vi "VI Linearisierung v2.vi"() -> ()   [LabVIEW 2020, in "Linearisierung v2.lvlib"] (continued)
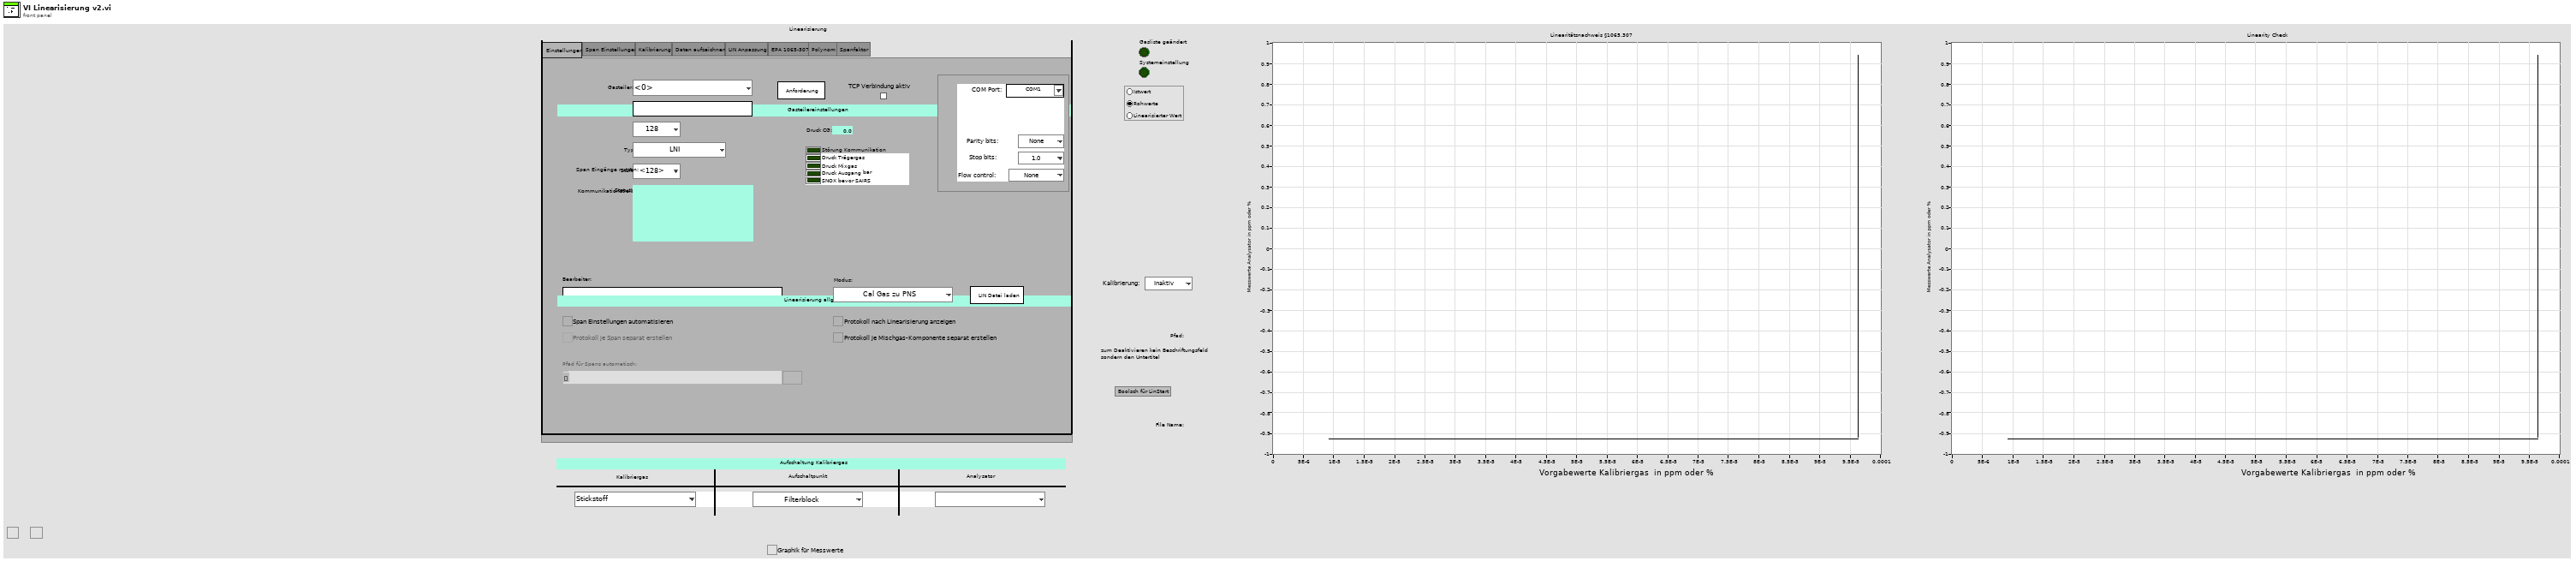
[diagram p1: front panel]
types:
  T1 = typedef "Checkbox(boolsch).ctl" = bool
  T2 = typedef "Linearisierung v2.lvlib/EPA Optionsfeld.ctl" = enum32{"Istwert", "Rohwert", "Linearisierter Wert"}
  T3 = typedef "EPA 1065.lvlib/T90 Test 1065-308.lvlib/Auswahl.ctl" = bool
  T4 = typedef "Button.ctl" = bool
  T5 = typedef "Linearisierung v2.lvlib/Kalibrieroption.ctl" = u16
  T6 = typedef "CalGas Aufschaltung.lvlib/Aufschaltung CalGas_ANZEIGE.ctl" = cluster{"Kalibriergas":T7, "Aufschaltpunkt":T7, "Analysator":T7}
  T7 = typedef "Auswahlfeld.ctl" = u16
  T8 = enum32{"Einstellungen", "Span Einstellungen", "HovaCAL Interface", "Kalibrierung", "Daten aufzeichnen", "LIN Anpassung", "EPA 1065-307", "Polynomkoeffizienten", "HovaCal Einstellungen", "Spanfaktor"}
  T9 = typedef "Pfad-Eingabefeld.ctl" = path
  T10 = typedef "CalGas Aufschaltung.lvlib/Lin Modus.ctl" = u16
  T11 = typedef "System Einstellungen V2.lvlib/Gasteiler Auswahl.ctl" = u16
  T12 = typedef "String - Eingabefeld.ctl" = string
  T13 = typedef "Linearisierung v2.lvlib/Gasteiler.lvlib/RS232.ctl" = cluster{"VISA Resource Name":refnum<visa-resource-name>, "Baud Rate":u32, "data bits":u16, "parity":u16, "stop bits":u16, "flow control":u16}
  T14 = typedef "Zahlen-Ausgabefeld.ctl" = sgl
  T15 = typedef "Linearisierung v2.lvlib/GasteilerType.ctl" = u16
  T16 = typedef "Linearisierung v2.lvlib/Gasteiler.lvlib/Gasteiler Stufen.ctl" = u16
  T17 = typedef "Linearisierung v2.lvlib/Gasteiler.lvlib/Gasteiler Fehler.ctl" = cluster{"Pressure carrier gas":bool, "Pressure diluted gas":bool, "Outlet Pressure":bool, "SNOX before SAIR":bool}
  T18 = enum32{"SPAN  1", "SPAN  2", "SPAN  3", "SPAN  4", "SPAN  5", "SPAN  6", "SPAN  7", "SPAN  8", "SPAN  9", "SPAN  10"}
  T19 = typedef "Linearisierung v2.lvlib/SpanEinstellungen.lvlib/SpanInletCluster.ctl" = cluster{"Span Inlet Active":T20, "Analysator":T21, "Konfig Gasflasche":T20, "Gasflasche":T22, "Gasflaschen Nr.:":string, "Ablaufdatum":timestamp, "Komponenten":T23, "Zeitdauer Stufen":sgl, "Max Fehler":sgl, "Anzahl Stufen":sgl, "Trägergas":T26, "zusätzliche Zeitdauer Erster Punkt":sgl}
  T20 = typedef "System Einstellungen V2.lvlib/Konfig Gasflasche.ctl" = bool
  T21 = typedef "System Einstellungen V2.lvlib/Analysatoren.ctl" = string
  T22 = typedef "System Einstellungen V2.lvlib/Gasflasche Auswahl.ctl" = u16
  T23 = typedef "Linearisierung v2.lvlib/SpanEinstellungen.lvlib/Komponentencluster mit Formel.ctl" = cluster{"Komponente 1":T24, "Komponente 2":T24, "Komponente 3":T24, "Komponente 4":T24, "Komponente 5":T24}
  T24 = typedef "Linearisierung v2.lvlib/SpanEinstellungen.lvlib/Komponentenauswahl mit Formel.ctl" = cluster{"Komponente:":u16, "Summenformel":T12, "Konzentration IST":dbl, "Einheit":T25, "Genauigkeit":dbl}
  T25 = typedef "Linearisierung v2.lvlib/SpanEinstellungen.lvlib/Einheit.ctl" = enum16{"ppm", "%"}
  T26 = typedef "System Einstellungen V2.lvlib/Traegergas.ctl" = string
  T27 = typedef "Linearisierung v2.lvlib/Gasteiler.lvlib/Stufen Tabelle.ctl" = string[][]
  T28 = typedef "Linearisierung v2.lvlib/Parameterkontrolle.ctl" = string[]
  T29 = typedef "Linearisierung v2.lvlib/Gasteiler.lvlib/HovaCAL_Interface.lvlib/Controls.lvlib/Pumpen Parameter Anzeige Eingabe.ctl" = cluster{"Reagent":T30, "concentratio mode":T31, "Molarity":dbl, "density":dbl, "syringe":dbl, "pumpe_a":dbl}[]
  T30 = typedef "Linearisierung v2.lvlib/Gasteiler.lvlib/HovaCAL_Interface.lvlib/Controls.lvlib/Reagent Anzeige.ctl" = i32
  T31 = typedef "Linearisierung v2.lvlib/Gasteiler.lvlib/HovaCAL_Interface.lvlib/Controls.lvlib/Pump Concentration Mode Anzeige.ctl" = i32
  T32 = typedef "Linearisierung v2.lvlib/Gasteiler.lvlib/HovaCAL_Interface.lvlib/Controls.lvlib/Pump state.ctl" = cluster{"Run":bool}
  T33 = typedef "Linearisierung v2.lvlib/Gasteiler.lvlib/HovaCAL_Interface.lvlib/Controls.lvlib/Flow Einstellung.ctl" = cluster{"HovaCAL Flow Input Cluster":dbl}
  T34 = typedef "Linearisierung v2.lvlib/Gasteiler.lvlib/HovaCAL_Interface.lvlib/Controls.lvlib/Flow Anzeige.ctl" = cluster{"Actual Flow":dbl}
  T35 = typedef "Linearisierung v2.lvlib/Gasteiler.lvlib/HovaCAL_Interface.lvlib/Controls.lvlib/Pumpen Parameter Anzeige.ctl" = cluster{"Reagent":T30, "concentratio mode":T31, "Molarity":dbl, "density":dbl, "syringe":dbl, "pumpe_a":dbl}[]
  T36 = typedef "Linearisierung v2.lvlib/Gasteiler.lvlib/HovaCAL_Interface.lvlib/Controls.lvlib/Pumpe Modus Anzeige.ctl" = cluster{"running?":bool, "dry mode":T37, "control mode":T38}
  T37 = typedef "Linearisierung v2.lvlib/Gasteiler.lvlib/HovaCAL_Interface.lvlib/Controls.lvlib/Pump Dry Mode Anzeige.ctl" = i32
  T38 = typedef "Linearisierung v2.lvlib/Gasteiler.lvlib/HovaCAL_Interface.lvlib/Controls.lvlib/Pump Control Mode Anzeige.ctl" = u32
  T39 = typedef "Linearisierung v2.lvlib/Gasteiler.lvlib/HovaCAL_Interface.lvlib/Controls.lvlib/Pumpe Status Anzeige.ctl" = cluster{"running?":bool, "Speed":dbl[]}
  T40 = typedef "Linearisierung v2.lvlib/Gasteiler.lvlib/HovaCAL_Interface.lvlib/Controls.lvlib/Pumpe MassenFluss Anzeige.ctl" = cluster{"reagent mf SP":dbl, "reagent mf":dbl, "water mf SP":dbl, "water mf":dbl, "water/reagent mf SP":dbl, "water/reagent mf":dbl}[]
  T41 = typedef "Linearisierung v2.lvlib/Gasteiler.lvlib/HovaCAL_Interface.lvlib/Controls.lvlib/Grenzen Anzeige.ctl" = cluster{"flow":dbl[], "temp":dbl[]}
  T42 = typedef "Linearisierung v2.lvlib/Gasteiler.lvlib/HovaCAL_Interface.lvlib/Controls.lvlib/Temp Sollwerte Anzeige.ctl" = dbl[]
  T43 = typedef "Linearisierung v2.lvlib/Gasteiler.lvlib/HovaCAL_Interface.lvlib/Controls.lvlib/Temp Ausgang Anzeige.ctl" = cluster{"temp 2":dbl, "temp":dbl, "humidity":dbl}[]
  T44 = typedef "Linearisierung v2.lvlib/Gasteiler.lvlib/HovaCAL_Interface.lvlib/Controls.lvlib/MFC Einstellungen.ctl" = cluster{"Input Concentration":dbl, "Output Setpoint":dbl}
  T45 = typedef "Linearisierung v2.lvlib/Gasteiler.lvlib/HovaCAL_Interface.lvlib/Controls.lvlib/MFC Output.ctl" = cluster{"output concentration":dbl, "output concentration dry":dbl, "flow actual":dbl, "flow expected":dbl}
  T46 = typedef "Linearisierung v2.lvlib/Gasteiler.lvlib/HovaCAL_Interface.lvlib/Controls.lvlib/MFC Konfiguration.ctl" = cluster{"MFC Gasauswahl":u16}
  T47 = typedef "Linearisierung v2.lvlib/Gasteiler.lvlib/HovaCAL_Interface.lvlib/Controls.lvlib/Pumpen Output.ctl" = cluster{"reagent conc":dbl, "reagent conc dry":dbl, "water conc":dbl, "water conc dry":dbl, "speed":dbl}
  T48 = typedef "String - Ausgabefeld.ctl" = string
  T49 = typedef "Linearisierung v2.lvlib/Gasnumber.ctl" = u8
  T50 = typedef "Linearisierung v2.lvlib/Gasteiler.lvlib/HovaCAL_Interface.lvlib/Controls.lvlib/Info Cluster Anzeige.ctl" = cluster{"device":string, "version":string, "number of mfc":i32, "number of pumps":i32, "number of temp controllers":i32, "number of mfs":i32, "number of balances":i32}
  T51 = typedef "Linearisierung v2.lvlib/Gasteiler.lvlib/HovaCAL_Interface.lvlib/Controls.lvlib/MFC Flow Anzeige.ctl" = cluster{"min flow":dbl, "max flow":dbl}[]
  T52 = typedef "Linearisierung v2.lvlib/Polynomkoeffizientenanzeige.ctl" = cluster{"Offset":dbl, "O.1":dbl, "O. 2":dbl, "O. 3":dbl, "O. 4":dbl}
  T53 = typedef "Linearisierung v2.lvlib/Ausgabetabelle.ctl" = string[][]
  T54 = typedef "Linearisierung v2.lvlib/Eingabetabelle.ctl" = string[][]
  T55 = typedef "Linearisierung v2.lvlib/Auswahl Polynom Ordnung.ctl" = enum16{"autom.", "raw", "actual", "1", "2", "3", "4"}
  T56 = typedef "Linearisierung v2.lvlib/LIN Ausgabetabelle.ctl" = string[][]
  T57 = typedef "Linearisierung v2.lvlib/AktivArray.ctl" = T58[]
  T58 = typedef "Linearisierung v2.lvlib/AktivButton.ctl" = bool
  T59 = typedef "Linearisierung v2.lvlib/Linearity verification 1065-307.lvlib/Condition.ctl" = u16
  T60 = typedef "Linearisierung v2.lvlib/EPA Ausgabetabelle.ctl" = string[][]
  T61 = typedef "Linearisierung v2.lvlib/Gasteiler.lvlib/HovaCal.lvlib/AutoLin Hovacal.ctl" = enum32{"Keine Auswahl", "Optionsauswahl 1", "Optionsauswahl 2"}
  T62 = typedef "Linearisierung v2.lvlib/Gasteiler.lvlib/HovaCal.lvlib/Dynamsiche_Werte.ctl" = cluster{"Durchfluss":dbl, "Drehzahl":dbl, "Wasserkonz.":dbl, "Ist - Temp":dbl, "Ist Konz 1":dbl, "Ist Konz 2":dbl}
  T63 = typedef "Linearisierung v2.lvlib/Gasteiler.lvlib/HovaCal.lvlib/Gase.ctl" = cluster{"Trägergas":u16, "Komponente 1":u16, "Komponente 2":u16}
  T64 = typedef "Linearisierung v2.lvlib/Gasteiler.lvlib/HovaCal.lvlib/Betriebsdaten.ctl" = cluster{"Gesamtdurchfluss":dbl, "Eingangskonzentration \nTrägergas":dbl, "Eingangskonzentration\nKomponente 1":dbl, "Eingangskonzentration \nKomponente 2":dbl, "Ausgangskonzentration \nKomponente 1 ":dbl, "Ausgangskonzentration\nKomponente 2":dbl, "l/min -> ml/min":bool, "N2 %->ppm":bool, "Komp1 ppm->%":bool, "Komp2ppm->%":bool, "Sollkomp1ppm->%":bool, "Sollkomp2ppm->%":bool}
  T65 = typedef "Linearisierung v2.lvlib/Gasteiler.lvlib/HovaCal.lvlib/Vaporizer.ctl" = cluster{"Pumpe Ein/Aus":dbl, "Wasser / Reagent":dbl, "Reagent dry / wet":dbl, "Reagent":dbl, "min. Temperatur\n160 °C":dbl, "Solltemperatur":dbl, "Wasserkonzentration\nSoll":dbl}
  T66 = enum8{"Enabled", "Disabled", "Disabled and Grayed Out"}
  T67 = typedef "Linearisierung v2.lvlib/SpanEinstellungen.lvlib/Aktion FGV SPAN Stufentabellen.ctl" = enum16{"lesen", "schreiben", "init"}
  T68 = typedef "Linearisierung v2.lvlib/Protokoll.lvlib/Aktion LIN Polynom Ordnung ode Aktiv Changes für Postprocessing.ctl" = enum16{"lesen", "schreiben", "init", "init initial"}
  T69 = cluster{"active SPAN Idx":i32, "active Component Index":i32}
  T70 = typedef "Linearisierung v2.lvlib/Protokoll.lvlib/Aktion LIN Polynom Ordnung je Komponente für Protokoll.ctl" = enum16{"lesen", "schreiben", "init", "schreiben viewonly", "init initial"}
  T71 = typedef "Linearisierung v2.lvlib/SpanEinstellungen.lvlib/Aktion FGV Post Processing.ctl" = enum16{"lesen", "set ref", "init", "reset", "enable", "disable", "filenames", "active", "comp", "filename index", "next", "first", "abort", "show", "same"}
  T72 = typedef "Linearisierung v2.lvlib/Gasteiler.lvlib/Aktion FGV Gasteilerliste laden.ctl" = enum16{"lesen", "laden", "speichern", "Liste erstellen", "Formel ändern", "Gas vereinzeln"}
  T73 = typedef "Linearisierung v2.lvlib/SpanEinstellungen.lvlib/Aktion FGV SPAN Verriegelung.ctl" = enum16{"lesen", "setrefs", "setcomp", "lock", "unlock", "Set Save EPA redirect", "Reset Save EPA redirect", "Set Postprocessing PDF", "Reset Postprocessing PDF", "Set Start Postprocessing PDF", "Reset Start Postprocessing PDF"}
  T74 = typedef "Linearisierung v2.lvlib/SpanEinstellungen.lvlib/Aktion FGV Spans abarbeiten.ctl" = enum16{"lesen", "idle", "start", "next", "comp", "init", "running", "abort"}
  T75 = typedef "Linearisierung v2.lvlib/SpanEinstellungen.lvlib/Aktion FGV SpanEinstellungen.ctl" = enum16{"lesen", "schreiben", "laden", "speichern", "RegisterRef", "automatisch", "init", "PDF Params", "Punkte umkehren"}
  T76 = typedef "System Einstellungen V2.lvlib/Aktion FGV Gasbottledefinition.ctl" = enum16{"lesen", "schreiben", "löschen", "laden", "speichern", "exportieren", "importieren"}
  T77 = typedef "Linearisierung v2.lvlib/SpanEinstellungen.lvlib/Aktion FGV Komponentenreferenz verwalten.ctl" = enum16{"Referenzen init", "lesen", "Referenzen schließen", "Ring beschreiben", "MFC fix Werte setzen"}
  T78 = typedef "FT-IR.lvlib/FGV FT-IR Gasliste Aktionen.ctl" = enum16{"lesen", "Gasliste FT-IR", "Gasliste ausgelesen", "laden", "speichern", "löschen"}
  T79 = typedef "Linearisierung v2.lvlib/Gasteiler.lvlib/HovaCAL_Interface.lvlib/Kommunikation.lvlib/Aktion_FGV_HovaCAL_Interface_Kommandos.ctl" = enum16{"lesen", "verarbeiten", "hinzufügen", "on top", "init", "sammeln", "freigeben", "connected"}
  T80 = typedef "Linearisierung v2.lvlib/Gasteiler.lvlib/HovaCAL_Interface.lvlib/Kommunikation.lvlib/Aktion_FGV_HovaCAL_Interface_GetData.ctl" = enum16{"lesen", "SystemInfo", "MFC Info", "actual Values", "Limits", "first contact", "reset after read"}
  T81 = typedef "Linearisierung v2.lvlib/Gasteiler.lvlib/HovaCAL_Interface.lvlib/Kommunikation.lvlib/Aktion_FGV_HovaCAL_Interface_SetData.ctl" = enum16{"lesen", "Konzentrationen", "Pumpen Parameter", "Pumpe Konzentration", "Pumpe run", "Temperaturen", "Fluss", "Limits", "init"}
  T82 = typedef "Linearisierung V2.lvlib/Aktion FGV Rohmesswerte sammeln.ctl" = enum16{"lesen", "schreiben", "löschen", "Sollwert HovaCal"}
  T83 = typedef "Linearisierung v2.lvlib/Aktion FGV Stoerungen sammeln und auswerten.ctl" = enum16{"init", "lesen", "error", "prüfen", "reset error", "abbrechen", "fortsetzen", "neustart", "Bedientasten reset"}
  T84 = typedef "Linearisierung v2.lvlib/Gasteiler.lvlib/Aktionen FGV Gasteiler Daten.ctl" = enum16{"lesen", "Gasteiler Daten", "Seriellen Param.", "MB-Endwert", "laden", "speichern", "Anforderung", "TCP", "Aufzeichnung Start"}
  T85 = typedef "FT-IR.lvlib/Spanfaktor.lvlib/Aktion FGV Span.ctl" = enum16{"lesen", "Span", "Seite aktiv", "Offset", "FGV aktualisiert", "Aktualisierung aufheben"}
  T86 = typedef "CalGas Aufschaltung.lvlib/FGV CalGas Aktionen.ctl" = enum16{"lesen", "Analysator Auswahl", "Def.CalGas", "Aufschaltung CalGas", "laden", "speichern", "KAL extrahieren"}
  T87 = typedef "Linearisierung v2.lvlib/LinV2 Registerkarten.ctl" = enum32{"Einstellungen", "HovaCAL Interface", "Kalibrierung", "Daten aufzeichnen", "LIN Anpassung", "EPA 1065-307", "Polynomkoeffizienten", "HovaCal Einstellungen", "Spanfaktor"}
  T88 = typedef "Linearisierung v2.lvlib/Gasteiler.lvlib/HovaCal.lvlib/Aktion_FGV_Betriebsdaten.ctl" = enum16{"Lesen", "Sollwerte schreiben", "Sollwerte lesen", "Gase schreiben", "Gase lesen", "Dynamische Werte", "GaseRef", "Gase aendern"}
  T89 = typedef "Linearisierung v2.lvlib/Gasteiler.lvlib/Gasteiler Type.ctl" = enum16{"LNI Digital", "LNI Analoge", "AVL GDU ", "Horiba GDC", "HovaCal"}
  T90 = typedef "Linearisierung v2.lvlib/Aktion Lin Daten aufarbeiten.ctl" = enum16{"lesen", "Protkolldaten", "speichern", "laden", "EPA auswerten", "Tabelle schreiben", "Lin auswerten", "Tab init", "Stufentabelle", "EPA aktiviert", "Nachbehandlung laden", "Tabelle löschen", "Istwerte löschen", "Zeile löschen", "Zeile einfügen", "LIN aktiviert", "LIN/EPA aktiv laden", "EGAK Tab", "LIN übernehmen", "Tab init ohne Stufen"}
  T91 = typedef "Linearisierung v2.lvlib/Gasteiler.lvlib/HovaCAL_Interface.lvlib/Kommunikation.lvlib/Aktion FGV HovaCAL Interface Autolin.ctl" = enum16{"lesen", "schreiben", "MFC Komponente fix setzen", "init"}
  T92 = typedef "Linearisierung v2.lvlib/Gasteiler.lvlib/Aktion FGV Daten Abholung uebergebenctl.ctl" = enum16{"lesen", "schreiben", "Anzeigebit löschen", "Status hinzufügen"}
  T93 = typedef "Linearisierung v2.lvlib/Gasteiler.lvlib/Aktion FGV Gasteiler Korrektur.ctl" = enum16{"lesen", "schreiben", "laden", "speichern", "B-nr und Gültig", "Gasteilernr.", "Vereinzeln", "aktiv"}
  T94 = typedef "Linearisierung v2.lvlib/Aktionen Polynom Daten speichern.ctl" = enum16{"lesen", "laden", "speichern", "schreiben", "schreiben alle", "Liste erstellen", "aktivieren", "deaktivieren", "aktiv abfragen"}
  T95 = typedef "Linearisierung v2.lvlib/Gasteiler.lvlib/HovaCal.lvlib/Aktion_FGV_Kom.ctl" = enum16{"Initialisieren", "Betriebsparameter", "Gase", "Vaporizer", "Dynamische Werte", "Beenden", "Com ändern", "Gase init"}
  T96 = typedef "Linearisierung v2.lvlib/Gasteiler.lvlib/HovaCAL_Interface.lvlib/Kommunikation.lvlib/Aktion_FGV_HovaCAL_Interface_Kommunikation.ctl" = enum16{"Initialisieren", "Set Konzentrationen", "Set Gase", "Set Limits", "Get Dynamische Werte", "Beenden", "Com ändern", "Get Gase init", "Pause", "Get Gasteiler Infos", "Get MFC Infos", "Set Pumpen Parameter", "Set Pumpe Konzenration", "Set Pumpe run", "Set Temperaturen", "Set Fluss", "Get Gase", "Get Limits", "Get Dynamische Werte 1", "Get Dynamische Werte 2"}
  T97 = typedef "PDF Interface.lvlib/PDF Interface Helper.lvlib/PDFResultPictures.ctl" = cluster{"Yes Ctl Refnum":refnum<vi>, "No Ctl Refnum":refnum<vi>}
  T98 = typedef "Sprachverwaltung.lvlib/FGV Aktion Tabelle zerlegen.ctl" = enum16{"laden", "vereinzeln", "speichern"}
  T99 = typedef "FT-IR.lvlib/Aktionen EVID-Codes.ctl" = enum16{"lesen", "setzen", "laden", "speichern", "1Hz/5Hz", "Smoothing", "Rolling Average"}
  T100 = typedef "LVRowAndColumnTypeDef.ctl" = cluster{"Row":i32, "Column":i32}
  T101 = cluster{"File Name LIN":refnum<vi>, "EPA Filename":refnum<vi>}
  T102 = cluster{"LIN Filename override":refnum<vi>, "EPA Filename override":refnum<vi>}
  T103 = cluster{"Spanfactor":refnum<vi>, "Offset":refnum<vi>, "Polynom":refnum<vi>}
  T104 = cluster{"Hauptregisterkarte":refnum<vi>, "SpanRegister":refnum<vi>}
  T105 = typedef "System Einstellungen V2.lvlib/Gasflasche gesamt.ctl" = cluster{"Gasflasche":T106, "Trägergas":T26, "Komponenten":T107[]}
  T106 = typedef "System Einstellungen V2.lvlib/Gasflasche.ctl" = cluster{"Gasname für die Auswahl":string, "Chargennummer":string, "Ablaufdatum":timestamp}
  T107 = typedef "System Einstellungen V2.lvlib/Gasflaschenkomponente.ctl" = cluster{"Gasauswahl":string, "Konzentration IST":dbl, "Einheit":string, "Genauigkeit":dbl}
  T108 = typedef "Linearisierung v2.lvlib/SpanEinstellungen.lvlib/PDF Optionen.ctl" = cluster{"PDF Einzelseiten Komponenten":bool, "PDF Einzelseiten Span":bool, "PDF Deckblatt":bool, "PDF öffnen":bool, "Graphik für Messwerte":bool}
  T109 = cluster{"Punkte umkehren":bool[], "PDF Optionen":T108}
  T110 = cluster{"Polynom-Ordnung":refnum<vi>, "Spanfactor LIN":refnum<vi>, "Offset LIN":refnum<vi>, "Polynomkoeffizienten":refnum<vi>}
  T111 = cluster{refnum<vi>[], refnum<vi>[], cluster{"Spanfactor":refnum<vi>, "Offset":refnum<vi>, "Polynom":refnum<vi>}, cluster{"Polynom-Ordnung":refnum<vi>, "Spanfactor LIN":refnum<vi>, "Offset LIN":refnum<vi>, "Polynomkoeffizienten":refnum<vi>}, "EPA Optionsfeld":refnum<vi>}
  T112 = cluster{"passive Komponente:":refnum<vi>, "post processing":refnum<vi>, "post processing done":refnum<vi>, "post processing PDFs":refnum<vi>}
  T113 = cluster{"post processing":refnum<vi>, "post processing done":refnum<vi>, "post processing PDFs":refnum<vi>}
  T114 = cluster{"System Cluster":refnum<vi>, "MFC Flow Cluster":refnum<vi>}
  T115 = cluster{refnum<vi>[], "Cluster.Temp Cluster":refnum<vi>, "Cluster.PumpModeGeneral-Cluster":refnum<vi>, refnum<vi>[], "Cluster.Flow Output Cluster (Ausgang)":refnum<vi>, "Cluster.Pump MassFlow-Cluster":refnum<vi>, "Cluster.PumpModeGeneral-Cluster 2":refnum<vi>}
  T116 = cluster{"HovaCAL Limits Cluster":refnum<vi>, "HovaCAL SetPumpMode":refnum<vi>, "HovaCAL Cluster.PumpModeGeneral":refnum<vi>, "HovaCAL SetPumpMode-Cluster":refnum<vi>, "HovaCAL Flow Input Cluster":refnum<vi>, refnum<vi>[], "HovaCAL Temperature":refnum<vi>, refnum<vi>[], "HovaCAL AutoLin MFC":refnum<vi>, refnum<vi>[]}
  T117 = typedef "Linearisierung v2.lvlib/Gasteiler.lvlib/HovaCAL_Interface.lvlib/Controls.lvlib/Info Cluster.ctl" = cluster{"device":string, "version":string, "number of mfc":i32, "number of pumps":i32, "number of temp controllers":i32, "number of mfs":i32, "number of balances":i32}
  T118 = typedef "Linearisierung v2.lvlib/Gasteiler.lvlib/Gasteiler Daten.ctl" = cluster{"Gasteiler":T12, "Gasteiler Stufen":T16, "Gasteiler Type":T15, "Konfig Gasteiler":T11, "Gasteiler Span Eingänge":u16}
  T119 = typedef "Linearisierung v2.lvlib/Lin-Polynom Daten.ctl" = cluster{"Messgerät":string, "Kalibrator (Gasteiler)":string, "Bearbeiter/in":string, "Komponente":string, "Zeitstempel":timestamp, "F_max gefordert (%)":sgl, "F_max in %":sgl, "F_max in ppm":sgl, "Vorschlag Ordnung":i32, "Polynom OK":bool, "Polynomkoeff.":dbl[], "Prüfgas Konzentration":dbl, "Pfad EPA":string, "Pfad_LIN":string, "Gasnummer:":u8, "Komponentenauswahl":T120, "Verdünnungsgas":T121, "Zeitdauer Stufe":T122, "Anzahl Stufen":T122, "F_max in % EPA":sgl, "F_max in ppm EPA":sgl, "F_max in % LIN":sgl, "F_max in ppm LIN":sgl, "Punkte umkehren":bool, "EPA Optionsfeld":T2, "Autolin Hovacal":T61, "Spanfactors":sgl[], "Kalibrierauswahl":T5, "Conditions:":T59, "Gasflaschen Nr.:":string, "Bottle Accuracy":dbl, "Konfig Gasflasche":T20, "Gasflasche":T22, "HovaCAL Flow AutoLin":T33, "MFC Output":T32, "Gas Ablaufdatum":timestamp, "Lin Modus":T10, "zusätzliche Zeitdauer Erster Punkt":sgl, "Offsets":sgl[]}
  T120 = typedef "Linearisierung v2.lvlib/KomponentenArray.ctl" = cluster{"Komponente:":T7, "Konzentration":dbl}[]
  T121 = typedef "Linearisierung v2.lvlib/Gasteiler.lvlib/Prüfgas in.ctl" = u16
  T122 = typedef "Zahlen-Eingabefeld.ctl" = sgl
  T123 = typedef "CalGas Aufschaltung.lvlib/Definition CalGas Anzeige.ctl" = cluster{"Namen":T124, "Werte":T125, "Werte 2":T125, "Einheit":T126, "Messbereiche":T127}
  T124 = typedef "CalGas Aufschaltung.lvlib/CalGas-Namen.ctl" = cluster{"Name":T12, "Name 2":T12, "Name 3":T12, "Name 4":T12, "Name 5":T12, "Name 6":T12, "Name 7":T12, "Name 8":T12, "Name 9":T12, "Name 10":T12, "Name 11":T12, "Name 12":T12}
  T125 = typedef "CalGas Aufschaltung.lvlib/CalGas-Werte.ctl" = cluster{"Konzentration 1":T122, "Konzentration 2":T122, "Konzentration 3":T122, "Konzentration 4":T122, "Konzentration 5":T122, "Konzentration 6":T122, "Konzentration 7":T122, "Konzentration 8":T122, "Konzentration 9":T122, "Konzentration 10":T122, "Konzentration 11":T122, "Konzentration 12":T122}
  T126 = typedef "CalGas Aufschaltung.lvlib/CalGas-Einheit.ctl" = cluster{"Einheit 1":T7, "Einheit 2":T7, "Einheit 3":T7, "Einheit 4":T7, "Einheit 5":T7, "Einheit 6":T7, "Einheit 7":T7, "Einheit 8":T7, "Einheit 9":T7, "Einheit 10":T7, "Einheit 11":T7, "Einheit 12":T7}
  T127 = typedef "CalGas Aufschaltung.lvlib/CalGas-Messbereiche.ctl" = cluster{"Messbereich 1":T7, "Messbereich 2":T7, "Messbereich 3":T7, "Messbereich 4":T7, "Messbereich 5":T7, "Messbereich 6":T7, "Messbereich 7":T7, "Messbereich 8":T7, "Messbereich 9":T7, "Messbereich 10":T7, "Messbereich 11":T7, "Messbereich 12":T7}
  T128 = cluster{"Aktive":bool, "IP-Adresse":string, "Port":u16}
  T129 = typedef "AK-Schnittstelle.lvlib/AK Seriell.lvlib/Serielle Parameter.ctl" = cluster{"VISA resource name":refnum<visa-resource-name>, "baud rate":u32, "data bits":u16, "parity":u16, "stop bits":u16, "flow control":u16}
  T130 = cluster{"PDF single pages Components":refnum<vi>, "PDF single pages Span":refnum<vi>, "PDF Deckblatt":refnum<vi>, "PDF öffnen":refnum<vi>}
  T131 = typedef "CalGas Aufschaltung.lvlib/Aufschaltung CalGas.ctl" = cluster{"Kalibriergas":T7, "Aufschaltpunkt":T132, "Analysator":T133}
  T132 = typedef "CalGas Aufschaltung.lvlib/Auswahl Aufschaltpunkt.ctl" = enum16{"über Filterblock", "Analysator direkt", "über PNS", "Entnahme", "Gasdivider"}
  T133 = typedef "CalGas Aufschaltung.lvlib/Auswahl Analysator.ctl" = enum16{"FT-IR", "FID", "PMA", "PMA/FID/FT-IR"}
  T134 = typedef "EPA 1065.lvlib/Aktion Test Status.ctl" = enum16{"init", "lesen", "prüfen", "Interference 366", "Interference 375", "Chiller läuft", "Drift läuft", "Pre Test läuft", "FID Optimization läuft", "FID Interference läuft", "HovaCAL Interference", "LinV2"}
  T135 = cluster{"STARTEN":refnum<vi>, "Abbrechen (Eingang)":refnum<vi>, "FORTSETZEN":refnum<vi>, "Speichern LIN":refnum<vi>}
  T136 = typedef "EPA 1065.lvlib/Aktion Wertaenderung Gasliste.ctl" = enum16{"Init", "lesen", "Gasliste geändert", "ARN inaktiv", "LEAK inaktiv", "Interference 366 inaktiv", "T90 inaktiv", "Interference 375 inaktiv", "Chiller inaktiv", "FID O2 inaktiv", "FID Opti inaktiv", "Drift inaktiv", "Pre Test inaktiv", "LinV2 inaktiv", "HovaCAL Interference inaktiv"}
  T137 = typedef "Linearisierung v2.lvlib/Gasteiler.lvlib/AK Komm Gasteiler.lvlib/Aktionen AK Komm.ctl" = enum16{"lesen", "initialisieren", "beenden", "Status", "SMAN", "SREM", "STBY", "ASTF", "ASTZ", "SLST", "AGAT", "EGAK", "AGAK", "AKAK", "ADRU", "SKOP", "SVSA", "SVSZ", "SONO", "SAIR", "SNOX", "ANOX", "SSPL", "SRUC", "SLIN", "ALST", "ETYP", "SVIO", "LCYL", "CCYL", "DCYL", "SCYL", "GCYL", "DRGV", "DRDC"}
  T138 = typedef "Linearisierung v2.lvlib/Gasteiler.lvlib/AK Komm Gasteiler.lvlib/Alter Gasteiler.lvlib/Aktionen AK Komm_ALT.ctl" = enum16{"lesen", "initialisieren", "beenden", "SRES", "STBY", "SREM", "SMAN", "SLIN", "SLCH", "SLST", "SSPL", "AGAT", "ALST", "ASTZ", "ASTF", "AGAK", "EGAK"}
  T139 = typedef "Linearisierung v2.lvlib/Gasteiler.lvlib/Horiba GDC.lvlib/Aktion Befehl.ctl" = enum16{"lesen", "initialisieren", "Beenden", "Standby", "GD/CC", "Info", "Flow", "Alarm", "GD parameter", "GD point", "Durchfluss", "Spuelen1", "Spuelen1 On", "Spuelen1Off", "Spuelen2", "Ventil-Abfrage", "Reset"}
  T140 = typedef "Passwort.lvlib/FGV Passwort Aktion.ctl" = enum16{"prüfen", "setzen", "Initialisieren", "PW speichern", "lesen", "PW Änderung"}
  T141 = typedef "Linearisierung v2.lvlib/Gasteiler.lvlib/HovaCAL_Interface.lvlib/Kommunikation.lvlib/Aktion_FGV_HovaCAL_Interface_Gasliste.ctl" = enum16{"lesen", "setzen", "erstellen"}
  T142 = typedef "System Einstellungen V2.lvlib/Aktion FGV SystemEinstellungenV2.ctl" = enum16{"lesen", "Analysatoren schreiben", "Analysator ändern", "Analysatoren löschen", "laden", "speichern", "Untertitel", "Analysatoren", "Neue Analysatoren", "Gasteiler schreiben", "Gasteiler ändern", "Gasteiler löschen", "Gasteiler", "Gasteiler exportieren", "Gasteiler importieren"}
  T143 = typedef "Funktionstasten.lvlib/Zustaende.ctl" = enum16{"Standby", "Pause", "Eco", "Messen", "Kalibrieren", "Spülen Filter", "Spülen Leitung", "Umgebungsluft", "0-Gas", "Cal-Gas", "CG zu PNS", "-------------", "Init 1", "Init 2", "Init 3", "Init 4", "Messen vorbereiten", "Messen durchführen", "Exit"}
  T144 = typedef "Funktionstasten.lvlib/Funktionstasten-Aktion.ctl" = enum16{"Initialisieren", "Zustand setzen", "Taste gedrückt", "Fehler speichern", "Lesen", "Manuell", "Remote", "Bitparallel", "Samplepoint", "Zeit Prüfen", "reset Umschalten"}
  T145 = typedef "Auto Kalibrieren.lvlib/Aktion FGV Autokal GT.ctl" = enum16{"lesen", "Autokal GT", "Referenz Start"}
  T146 = typedef "ABB-EL3000.lvlib/PMA.lvlib/Kalibrieren.lvlib/Kalibrierung O2.ctl" = enum16{"Nullpunkt O2", "Endpunkt O2"}
  T147 = typedef "ABB-EL3000.lvlib/FID.lvlib/FID Kalibrierung.lvlib/FID Kalibrieren.ctl" = enum16{"CH4 Nullpunkt", "THC Nullpunkt", "NMHC Nullpunkt", "CH4 Endpunkt", "THC Endpunkt", "NMHC Endpunkt"}
  T148 = enum16{"Lesen", "Vaporizer lesen", "Vaporizer schreiben"}
  T149 = typedef "Linearisierung v2.lvlib/Protokoll.lvlib/Aktion EPA Polynom Ordnung je Komponente für Protokoll.ctl" = enum16{"lesen", "schreiben", "init", "init initial"}
  T150 = typedef "Linearisierung v2.lvlib/Linearity verification 1065-307.lvlib/Aktion FGV Auswertung sammeln.ctl" = enum16{"lesen", "Auswertung", "löschen"}
  T151 = cluster{"first contact in":bool, "first actual values in ":bool}
  T152 = typedef "Linearisierung v2.lvlib/SpanEinstellungen.lvlib/GD Abfrage Referenzen.ctl" = cluster{"Stufen Tabelle Array":refnum<vi>[], "auto Scan Points":refnum<vi>[], "Punkte umkehren":refnum<vi>[], "Parameterkontrolle Array":refnum<vi>[], "Eingabetabelle":refnum<vi>, "Ausgabetabelle":refnum<vi>, "Anforderung":refnum<vi>, "Status Str Referenz":refnum<vi>, "Prüfgasnamen Array":refnum<vi>[]}
  T153 = typedef "Linearisierung v2.lvlib/Aktion FGV GD Status Anzeige.ctl" = enum16{"lesen", "schreiben", "hinzufügen"}
  T154 = typedef "Linearisierung v2.lvlib/SpanEinstellungen.lvlib/Aktion FGV GD Errors sammeln.ctl" = enum16{"lesen", "init", "GD Infos sammeln", "Kalibrierinfos sammeln", "Test Data", "GD Infos selektiv sammeln"}
  T155 = typedef "Linearisierung v2.lvlib/SpanEinstellungen.lvlib/Postprocessing_Running_Indices.ctl" = cluster{"active postprocessing SPAN":i32, "active postprocessing SPAN Component":i32, "active postprocessing index":i32}
  T156 = typedef "Linearisierung v2.lvlib/LIN ErrorCluster.ctl" = cluster{"Störung Kommunikation":bool, "Pressure carrier gas":bool, "Pressure diluted gas":bool, "Outlet Pressure":bool, "SNOX before SAIR":bool, "Störung Gasteiler":bool}
  T157 = cluster{"Stufen Tabellen in":string[][][], "EGAK":T26[], "AGAK":string[]}
  T158 = typedef "eventsource.ctl" = u32
  T159 = typedef "lveventtype.ctl" = enum32{"Null", "Timeout", "Annotation Menu Selection", "Annotation Menu Selection?", "App Instance Close", "App Instance Close?", "Autoscale Range Change", "Bookmark Info Change", "Cell Edit", "Cell Edit?", "Cursor Grab", "Cursor Grab?", "Cursor Menu Selection", "Cursor Menu Selection?", "Cursor Move", "Cursor Release", "Data Change", "Direction Change", "Display State Change", "Drag Ended", "Drag Enter", "Drag Leave", "Drag Over", "Drag Source Update", "Drag Starting", "Drag Starting?", "Drop", "Exec State Change", "Key Down", "Key Down?", "Key Repeat", "Key Repeat?", "Key Up", "Listbox Double Click", "Menu Activation?", "Menu Selection (App)", "Menu Selection? (App)", "Menu Selection (User)", "Mouse Down", "Mouse Down?", "Mouse Enter", "Mouse Leave", "Mouse Move", "Mouse Up", "Mouse Wheel", "NI Security User Change (App)", "Pane Size", "Panel Close", "Panel Close?", "Panel Resize", "Plot Attribute Change", "Scale Range Change", "Shortcut Menu Activation?", "Shortcut Menu Selection (App)", "Shortcut Menu Selection? (App)", "Shortcut Menu Selection (User)", "Tree Double Click", "Tree Drag", "Tree Drag?", "Tree Drop", "Tree Drop?", "Tree Item Close", "Tree Item Close?", "Tree Item Open", "Tree Item Open?", "User Event", "Value Change"}
  T160 = typedef "Verwaltung - cRIO.lvlib/Analog Eingaenge.ctl" = cluster{"AI0: Durchfluss FT-IR":sgl, "AI1: Druck Ausgang":sgl, "AI2: Umgebungsdruck":sgl, "AI3: Druck FT-IR":sgl, "AI4: Druck CalGas":sgl, "AI5: Reserve":sgl, "AI6: Reserve":sgl, "AI7: Reserve":sgl, "Rohwert Durchfluss FT-IR":sgl, "Rohwert Druck Ausgang":sgl, "Rohwert Umgebungsdruck":sgl, "Rohwert Druck FT-IR":sgl, "Rohwert Druck CalGas":sgl, "Rohwert AI5":sgl, "Rohwert AI6":sgl, "Rohwert AI7":sgl, "Rohwert Diffdruck mbar FTIR":sgl}
  T161 = typedef "Linearisierung v2.lvlib/Gasteiler.lvlib/HovaCAL_Interface.lvlib/Controls.lvlib/Pump Concentration Mode.ctl" = i32
  T162 = typedef "Linearisierung v2.lvlib/Gasteiler.lvlib/HovaCAL_Interface.lvlib/Controls.lvlib/Reagent.ctl" = i32
  T163 = cluster{"concentratio mode":T161, "Reagent":T162, "Molarity":dbl, "density":dbl, "syringe":dbl, "pumpe_a":dbl}[]
  T164 = typedef "Linearisierung v2.lvlib/Gasteiler.lvlib/HovaCAL_Interface.lvlib/Controls.lvlib/Pump Dry Mode.ctl" = i32
  T165 = typedef "Linearisierung v2.lvlib/Gasteiler.lvlib/HovaCAL_Interface.lvlib/Controls.lvlib/Pump Control Mode.ctl" = u32
  T166 = cluster{"running?":bool, "dry mode":T164, "control mode":T165}
  T167 = typedef "Linearisierung v2.lvlib/Gasteiler.lvlib/HovaCAL_Interface.lvlib/Controls.lvlib/Pump Concentration.ctl" = cluster{"reagent conc SP":dbl, "water conc SP":dbl}
  T168 = cluster{"input concentration setpoint":dbl, "output concentration setpoint":dbl}[]
  T169 = cluster{"concentratio mode":T161, "Reagent":T162, "Molarity":dbl, "density":dbl, "syringe":dbl, "pump_a":dbl}[]
  T170 = cluster{"input concentration setpoint":dbl, "output concentration setpoint":dbl}
  T171 = cluster{"reagent mf SP":dbl, "reagent mf":dbl, "water mf SP":dbl, "water mf":dbl, "water/reagent mf SP":dbl, "water/reagent mf":dbl}[]
  T172 = cluster{"reagent conc":dbl, "reagent conc dry":dbl, "water conc":dbl, "water conc dry":dbl, "speed":dbl}[]
  T173 = cluster{"temp SP":dbl, "temp":dbl, "humidity":dbl}[]
  T174 = cluster{"reagent conc":dbl, "reagent conc dry":dbl, "water conc":dbl, "water conc dry":dbl, "speed":dbl}
  T175 = cluster{"Einzelnes Polynom out[0]":dbl, "Einzelnes Polynom out[1]":dbl, "Einzelnes Polynom out[2]":dbl, "Einzelnes Polynom out[3]":dbl, "Einzelnes Polynom out[4]":dbl}
  T176 = typedef "LVRowAndColumnUnsignedTypeDef.ctl" = cluster{"Row":u32, "Column":u32}
  T177 = cluster{"Pressure carrier gas":bool, "Pressure diluted gas":bool, "Outlet Pressure":bool, bool}
  T178 = typedef "EPA 1065.lvlib/Aktive Tests Cluster.ctl" = cluster{"ANR läuft":bool, "T90 läuft":bool, "Leak läuft":bool, "Interference 366 läuft":bool, "Interference 375 läuft":bool, "Chiller läuft":bool, "FID Interference läuft":bool, "FID optimization läuft":bool, "Drift läuft":bool, "Pre-test läuft":bool, "HovaCAL Interference läuft":bool, "LinV2 läuft":bool}
  T179 = typedef "System Einstellungen V2.lvlib/Gasteiler.ctl" = cluster{"Gasteiler Name":string, "Gasteiler Type":string, "Gasteiler Seriennummer":string, "Gasteiler Letzte Wartung":timestamp}
  T180 = cluster{"GasteilerDefinitionsListe":T179[], "GasteilerDefinitionTextliste":string[][], "Gasteiler Strings And Values":cluster{"String":string, "Wert":string}[]}
  T181 = cluster{"Trägergas":bool, "Komponente 1":bool, "Komponente 2":bool}
  T182 = cluster{"Pumpe Ein/Aus":bool, "Wasser / Reagent":bool, "Reagent dry / wet":bool, "Reagent":bool, "min. Temperatur\n160 °C":bool, "Solltemperatur":bool, "Wasserkonzentration\nSoll":bool}
  T183 = cluster{"Gesamtdurchfluss":bool, "Eingangskonzentration \nTrägergas":bool, "Eingangskonzentration\nKomponente 1":bool, "Eingangskonzentration \nKomponente 2":bool, "Ausgangskonzentration \nKomponente 1 ":bool, "Ausgangskonzentration\nKomponente 2":bool, "l/min -> ml/min":bool, "N2 %->ppm":bool, "Komp1 ppm->%":bool, "Komp2ppm->%":bool, "Sollkomp1ppm->%":bool, "Sollkomp2ppm->%":bool}
  T184 = cluster{"Polynome[0]":dbl, "Polynome[1]":dbl, "Polynome[2]":dbl, "Polynome[3]":dbl, "Polynome[4]":dbl}
  T185 = cluster{"Polynomkoeff.[0]":dbl, "Polynomkoeff.[1]":dbl, "Polynomkoeff.[2]":dbl, "Polynomkoeff.[3]":dbl, "Polynomkoeff.[4]":dbl}
  T186 = typedef "Linearisierung v2.lvlib/SpanEinstellungen.lvlib/SpanComponentInfos-Cluster.ctl" = cluster{"SPAN Names":string[], "Component Infos":T187[], "GasBottleInfoArray":cluster{"Gasname für die Auswahl":string, "Chargennummer":string}[]}
  T187 = typedef "Linearisierung v2.lvlib/SpanEinstellungen.lvlib/ComponentInfos.ctl" = cluster{T48[], T12[], T48[]}
  T188 = cluster{"locked":bool, "Save EPA redirect":bool, "Postprocessing PDF":bool, "Start Postprocessing PDF":bool}
  T189 = cluster{"SPAN Idx out":i32, "first aktive Komponente":i32}
  T190 = cluster{"Bearbeiter/in":string, "Messgerät":string}
  T191 = cluster{"Komponente":string, i32, "Einheit in String":string}
  T192 = cluster{"PDF Optionen (Ausgang)":T108, "File Name LIN":T12, "Pfad Auto Lin":T9, "SPAN Idx out":i32, "first aktive Komponente":i32, bool, "LIN Filename override":T1}
  T193 = cluster{"EPA Ausgabetabelle ":string[][], "XY-Graph":cluster{dbl[], dbl[]}[], "LINVer Auswertung":string[][]}
  T194 = cluster{"LIN Ausgabetabelle ":string[][], "XY-Graph":cluster{dbl[], dbl[]}[], "Polynomkoeff.":cluster{"Polynomkoeff.[0]":sgl, "Polynomkoeff.[1]":sgl, "Polynomkoeff.[2]":sgl, "Polynomkoeff.[3]":sgl, "Polynomkoeff.[4]":sgl}}
  T195 = cluster{"Ausgabetabelle":T53, "Eingabetabelle behandelt":string[][]}
  T196 = typedef "Linearisierung v2.lvlib/SpanEinstellungen.lvlib/ErrorLogInfoCluster.ctl" = cluster{"Component Name":T48, "Gasflasche":T22, "last actice SPAN Idx out":i32, "Timestamp":string}
  T197 = cluster{"File Name LIN":string, "File Name EPA":string, "Deckblatt LIN":string, "Deckblatt EPA":string, "LIN TXT Datei Name":string}
  T198 = cluster{"Polynomkoeff.[0]":sgl, "Polynomkoeff.[1]":sgl, "Polynomkoeff.[2]":sgl, "Polynomkoeff.[3]":sgl, "Polynomkoeff.[4]":sgl}
  T199 = cluster{"Component":cluster{"Component Name":string, "Component":u8, "Component Unit":string}, "Daten aufzeichnen Offset Cluster":cluster{"Autorange Offsets":string, "Autorange Spanfactors":string, "Polynome":cluster{"Polynome[0]":dbl, "Polynome[1]":dbl, "Polynome[2]":dbl, "Polynome[3]":dbl, "Polynome[4]":dbl}}, "Lin Offset Cluster":cluster{"Autorange Offsets":string, "Autorange Spanfactors":string, "Polynome":cluster{"Polynome[0]":dbl, "Polynome[1]":dbl, "Polynome[2]":dbl, "Polynome[3]":dbl, "Polynome[4]":dbl}, "Polynom-Ordnung":T55}, "EPA Optionsfeld":T2}
  T200 = cluster{"PDF Optionen (Ausgang)":T108, "postprocess":bool, bool, "Pfad Auto Lin":T9, "File Name LIN":T12, "Pfad LIN":T9, "LIN Filename override":T1}
  T201 = cluster{"SpanComponentInfos-Cluster":T186, "Span_Name":string}
  T202 = cluster{"active postprocessing SPAN":i32, ".LIN Datei Pfad":path}
  T203 = cluster{"XY-Graph LIN 2":refnum<vi>, "XY-Graph EPA 2":refnum<vi>, "ResultPictures":T97, cluster{"File Name LIN":refnum<vi>, "EPA Filename":refnum<vi>}}
  T204 = typedef "Linearisierung v2.lvlib/SpanEinstellungen.lvlib/LIN Loading Setup Data.ctl" = cluster{"[Header]":string, "[Model]":string, "[active SPANs]":string, "[Analyser]":string, "[FT-IR_NOC_CTM_CTTW]":string, "[Recipie]":string, "[GasDivider]":string, "[GasBottle]":string, "[Polynomial]":string, "[SpanFactors]":string}
  T205 = typedef "Linearisierung v2.lvlib/SpanEinstellungen.lvlib/LIN Loading Errors.ctl" = cluster{"Rezept nicht ident":bool, "FT-IR nicht ident":bool, "FT-IR NOC CTM nicht ident":bool, "Gasliste nicht ident":bool, "aktive SPANs nicht ident":bool, "Polynom nicht ident":bool, "Span Faktoren nicht ident":bool}
  T206 = cluster{"[[LIN Polynom Settings]":string, "[[LIN Active]":string, "[[EPA Active]":string}
  T207 = cluster{"Label.Text":string, "Rezept nicht ident":bool}[]
  T208 = cluster{"GD DF":T20, "GD LNI old":T20, "GD Span Eingänge":u16}
  T209 = cluster{"manuelle Anforderung":bool, "show Message ":bool, "set Tables":bool, "set Tables":bool}
  T210 = cluster{"SPAN Index out":i32, "Component Index out":i32}
  T211 = cluster{"active SPAN Idx":i32, "Pfad .LIN Datei":T9}[]
  T212 = cluster{"active SPAN Idx":i32, "Pfad .LIN Datei":T9}
  T213 = cluster{"Index active SPAN":i32, "Component Idx":i32, u16}
  T214 = cluster{"TCP Verbindung aktiv":bool, string, "Port":u16}
  T215 = cluster{"manuelle Anforderung":bool, "show Message":bool, "set Tables":bool, "set Tables":bool}
  T216 = cluster{"Anzahl Stufen":sgl, "Trägergas":T26, "SPAN Idx out (Ausgang)":i32}
  T217 = cluster{"Komponente:":u16, "Konzentration IST":dbl}[]
  T218 = cluster{"Stufen Tabellen out":string[][][], "EGAK":T26[], "AGAK":string[]}
  T219 = cluster{"SPAN Idx out":i32, "Component Index out":i32}
  T220 = cluster{i32, cluster{"SPAN Idx out":i32, "Component Index out":i32}}
  T221 = cluster{bool, bool, "Gesamtkonzentration":dbl, "höchste Konzentration Teilkomponente":dbl}
  T222 = cluster{"SPAN Idx out (Ausgang)":i32, "Component Index out":i32}
  T223 = cluster{i32, cluster{"SPAN Idx out (Ausgang)":i32, "Component Index out":i32}}
  T224 = cluster{"MFC Komponenten Array":refnum<vi>[], "MFC fix + Array":refnum<vi>[]}
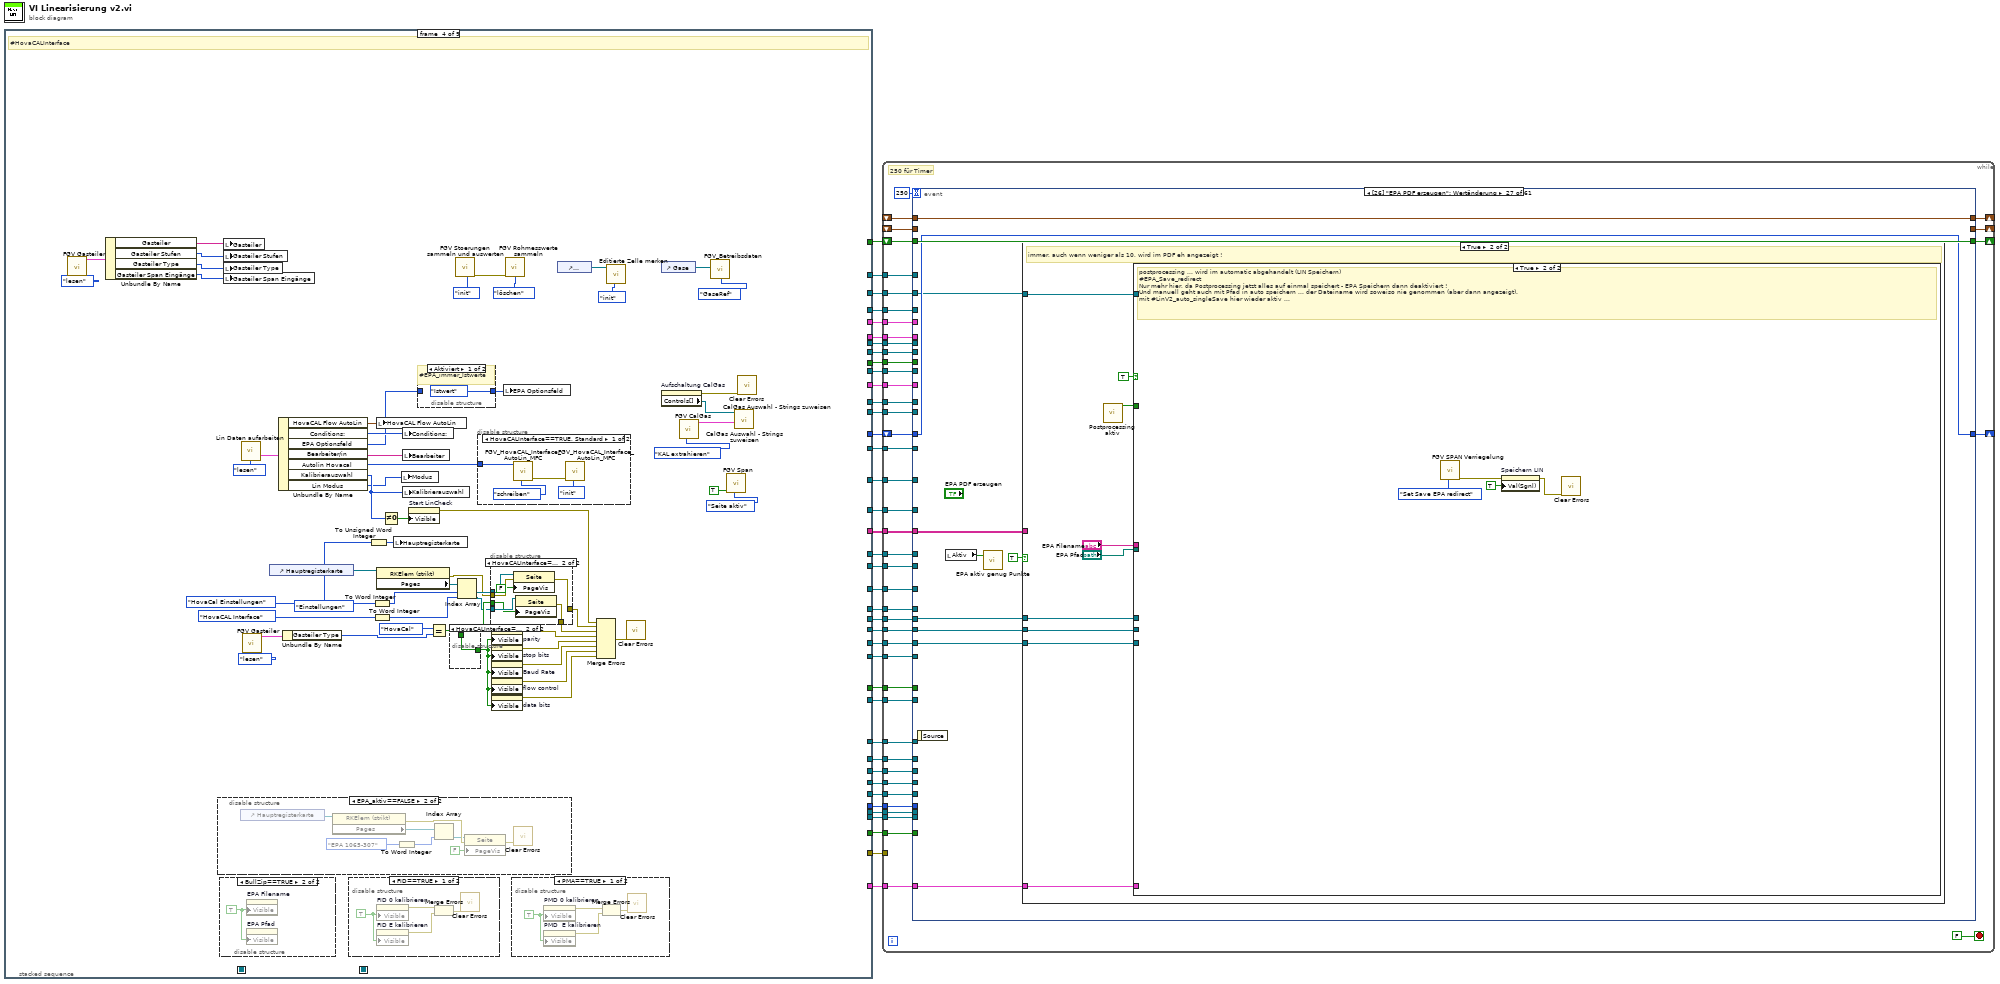
[diagram p0: block diagram]
diagram:
  n1 = stacked-sequence {
    seq-local: [w73 _ _ _ _ _ _ _ _] -> [_ w203 _ _ _ _ _ _ _]
    seq-local: [_ w168 _ _ _ _ _ _ _] -> [_ _ w339 _ _ _ _ _ _]
    tunnel: [_ _ _ _ _ w655 _ _ _] -> w39
    tunnel: [_ _ _ _ _ w665 _ _ _] -> w38
    tunnel: [_ _ _ _ w595 _ _ _ _] -> w37
    tunnel: [_ _ w373 _ _ _ _ _ _] -> w36
    tunnel: [_ w167 _ _ _ _ _ _ _] -> w35
    tunnel: [w107 _ _ _ _ _ _ _ _] -> w34
    tunnel: [w96 _ _ _ _ _ _ _ _] -> w33
    tunnel: [w85 _ _ _ _ _ _ _ _] -> w32
    tunnel: [w72 _ _ _ _ _ _ _ _] -> w31
    tunnel: [w73 _ _ _ _ _ _ _ _] -> w30
    tunnel: [_ _ _ _ _ w648 _ _ _] -> w29
    tunnel: [_ _ _ _ _ _ _ _ w684] -> w28
    tunnel: [_ _ _ _ w562 _ _ _ _] -> w27
    tunnel: [_ _ _ _ w563 _ _ _ _] -> w26
    tunnel: [_ _ _ _ w542 _ _ _ _] -> w25
    tunnel: [_ _ _ _ w559 _ _ _ _] -> w24
    tunnel: [w71 _ _ _ _ _ _ _ _] -> w23
    tunnel: [_ _ _ _ w547 _ _ _ _] -> w22
    tunnel: [_ _ _ _ w546 _ _ _ _] -> w21
    tunnel: [_ _ _ _ w545 _ _ _ _] -> w20
    tunnel: [_ _ _ _ w533 _ _ _ _] -> w19
    tunnel: [w50 _ _ _ _ _ _ _ _] -> w18
    tunnel: [_ _ _ _ _ _ _ _ w683] -> w17
    tunnel: [_ _ _ _ _ w645 _ _ _] -> w16
    tunnel: [_ _ _ _ _ _ _ _ w682] -> w15
    tunnel: [_ _ _ _ _ _ _ _ w681] -> w14
    tunnel: [_ _ _ _ _ _ _ _ w680] -> w13
    tunnel: [_ _ _ _ _ _ _ _ w679] -> w12
    tunnel: [_ w167 _ _ _ _ _ _ _] -> w11
    tunnel: [_ w166 _ _ _ _ _ _ _] -> w10
    tunnel: [_ _ w330 _ _ _ _ _ _] -> w9
    tunnel: [_ _ _ _ w520 _ _ _ _] -> w8
    tunnel: [w49 _ _ _ _ _ _ _ _] -> w7
    tunnel: [w48 _ _ _ _ _ _ _ _] -> w6
    tunnel: [w47 _ _ _ _ _ _ _ _] -> w5
    tunnel: [_ _ _ _ _ w641 _ _ _] -> w4
    tunnel: [w44 _ _ _ _ _ _ _ _] -> w3
    tunnel: [w43 _ _ _ _ _ _ _ _] -> w2
    tunnel: [w40 _ _ _ _ _ _ _ _] -> w1
    frame #0 {
      # "#Option10xSpanAuto"
      n2 = control-ref of="Dieses VI"() -> (w70:refnum<vi>)
      n3 = call "in Ursprung setzen.vi"("VI Referenz"=w70) -> ()  [unwired: 10 in, 1 out]
      n4 = control-ref of="Punkte umkehren"() -> (w74:refnum<vi>)
      n5 = control-ref of="Punkte umkehren 2"() -> (w59:refnum<vi>)
      n6 = control-ref of="Punkte umkehren 3"() -> (w58:refnum<vi>)
      n7 = control-ref of="Punkte umkehren 4"() -> (w57:refnum<vi>)
      n8 = control-ref of="Punkte umkehren 5"() -> (w56:refnum<vi>)
      n9 = control-ref of="Punkte umkehren 6"() -> (w55:refnum<vi>)
      n10 = control-ref of="Punkte umkehren 7"() -> (w54:refnum<vi>)
      n11 = control-ref of="Punkte umkehren 8"() -> (w53:refnum<vi>)
      n12 = control-ref of="Punkte umkehren 9"() -> (w52:refnum<vi>)
      n13 = control-ref of="Punkte umkehren 10"() -> (w51:refnum<vi>)
      n14 = control-ref of="PrüfgasName"() -> (w60:refnum<vi>)
